vi "USBCool.vi"() -> ()   [LabVIEW 2015]
panel:
  out "Set Gate Mode":u32
  out "Shut Down":u32
  out "Cooler OFF":u32
  out "Detector Y Pixels":i32
  out "Get Detector":u32
  out "Get Status":u32
  out "Get Temperature":u32
  out "Cooler ON":u32
  out "Set Exposure Time":u32
  out "Set Trigger Mode":u32
  out "Set Readout Mode":u32
  out "Set Acquisition Mode":u32
  out "Current Temperature":i32
  out "Set Temperature":u32
  in  "Temperature":i32
  out "Check Timings":u32
  out "Detector X Pixels":i32
  out "Status":u32
  out "Graphical Results":i32[](graph)
  out "Start Acquisition":u32
  out "Get Acquired Data":u32
  out "Calculated Exposure Value":sgl format="%.5f"
  in  "Exposure Time (secs)":sgl format="%.2f"
  out "Initialize":u32
  in  "Trigger":u32(ring) items=["Internal", "External"]
  # "Status"
  # "Return values"
  # "USB iStar COOL32at.VI"
  # "Acquisition Mode: Single Scan\nReadout Mode: Full Vertical Binning\nCools to desired temperature, acquires data and then brings the temperature up to 0 in a controlled way."
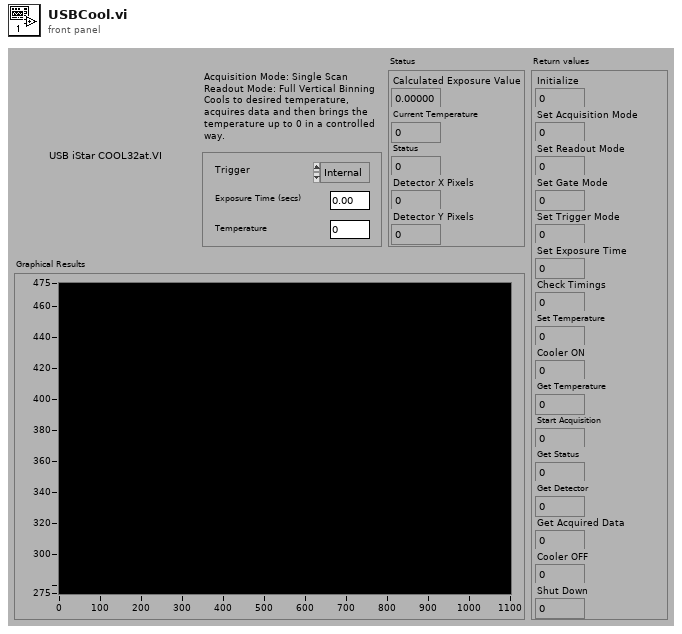
[diagram p1: front panel]
types:
  T1 = typedef "Error Code Enum typedef.ctl" = enum32{"N/A (0)", "DRV_ERROR_CODES", "DRV_SUCCESS", "DRV_VXDNOTINSTALLED", "DRV_ERROR_SCAN", "DRV_ERROR_CHECK_SUM", "DRV_ERROR_FILELOAD", "DRV_UNKNOWN_FUNC", "DRV_ERROR_VXD_INIT", "DRV_ERROR_ADDRESS", "DRV_ERROR_PAGELOCK", "DRV_ERROR_PAGEUNLOCK", "DRV_ERROR_BOARDTEST", "DRV_ERROR_ACK", "DRV_ERROR_UP_FIFO", "DRV_ERROR_PATTERN", "N/A (16)", "DRV_ACQUISITION_ERRORS", "DRV_ACQ_BUFFER", "DRV_ACQ_DOWNFIFO_FULL", "DRV_PROC_UNKONWN_INSTRUCTION", "DRV_ILLEGAL_OP_CODE", "DRV_KINETIC_TIME_NOT_MET", "DRV_ACCUM_TIME_NOT_MET", "DRV_NO_NEW_DATA", "N/A (25)", "DRV_SPOOLERROR", "N/A (27)", "N/A (28)", "N/A (29)", "N/A (30)", "N/A (31)", "N/A (32)", "DRV_TEMPERATURE_CODES", "DRV_TEMPERATURE_OFF", "DRV_TEMPERATURE_NOT_STABILIZED", "DRV_TEMPERATURE_STABILIZED", "DRV_TEMPERATURE_NOT_REACHED", "DRV_TEMPERATURE_OUT_RANGE", "DRV_TEMPERATURE_NOT_SUPPORTED", "DRV_TEMPERATURE_DRIFT", "N/A (41)", "N/A (42)", "N/A (43)", "N/A (44)", "N/A (45)", "N/A (46)", "N/A (47)", "N/A (48)", "DRV_GENERAL_ERRORS", "DRV_INVALID_AUX", "DRV_COF_NOTLOADED", "DRV_FPGAPROG", "DRV_FLEXERROR", "DRV_GPIBERROR", "N/A (55)", "N/A (56)", "N/A (57)", "N/A (58)", "N/A (59)", "N/A (60)", "N/A (61)", "N/A (62)", "N/A (63)", "DRV_DATATYPE", "DRV_DRIVER_ERRORS", "DRV_P1INVALID", "DRV_P2INVALID", "DRV_P3INVALID", "DRV_P4INVALID", "DRV_INIERROR", "DRV_COFERROR", "DRV_ACQUIRING", "DRV_IDLE", "DRV_TEMPCYCLE", "DRV_NOT_INITIALIZED", "DRV_P5INVALID", "DRV_P6INVALID", "DRV_INVALID_MODE", "DRV_INVALID_FILTER", "DRV_I2CERRORS", "DRV_I2CDEVNOTFOUND", "DRV_I2CTIMEOUT", "DRV_P7INVALID", "N/A (84)", "N/A (85)", "N/A (86)", "N/A (87)", "N/A (88)", "N/A (89)", "DRV_IOCERROR", "DRV_VRMVERSIONERROR"}
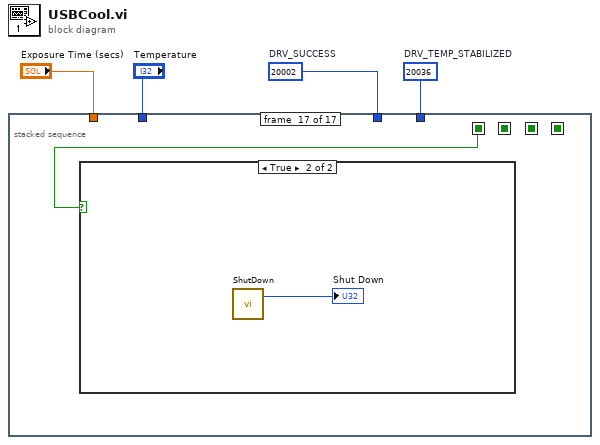
[diagram p0: block diagram]
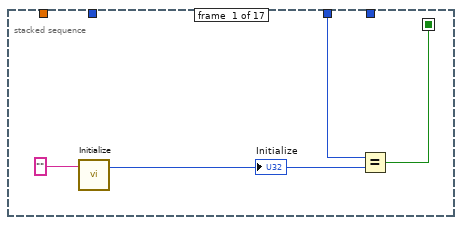
[diagram p2: hidden frame]
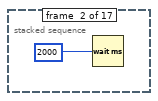
[diagram p3: hidden frame]
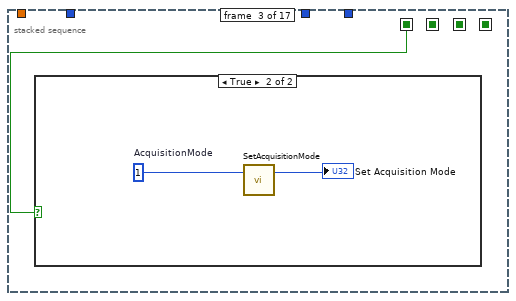
[diagram p4: hidden frame]
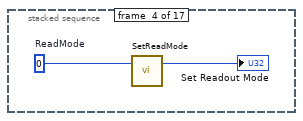
[diagram p6: hidden frame]
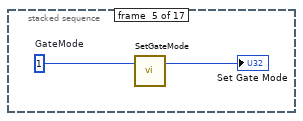
[diagram p7: hidden frame]
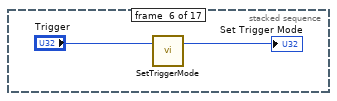
[diagram p8: hidden frame]
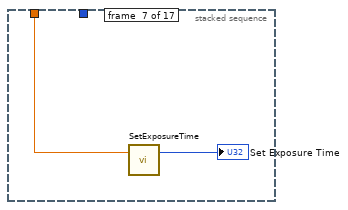
[diagram p9: hidden frame]
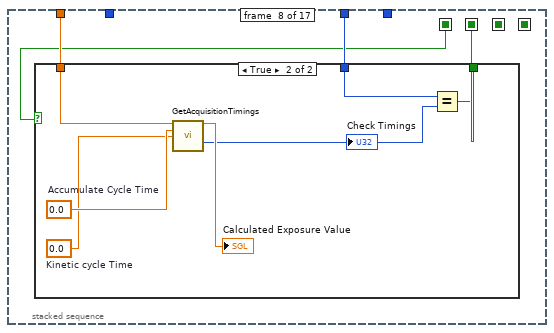
[diagram p10: hidden frame]
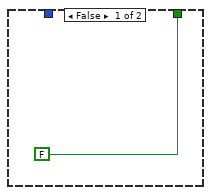
[diagram p11: hidden frame]
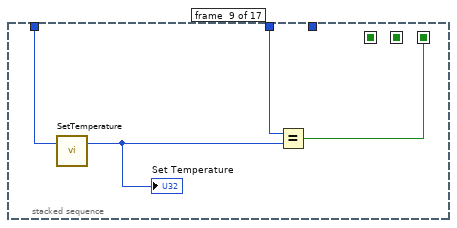
[diagram p12: hidden frame]
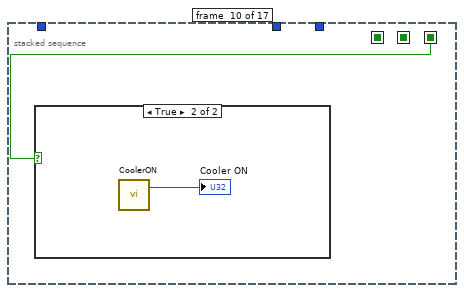
[diagram p13: hidden frame]
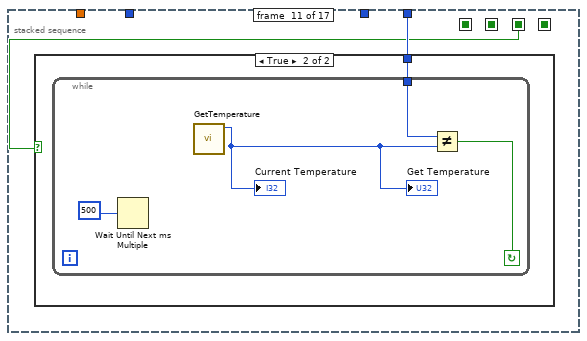
[diagram p15: hidden frame]
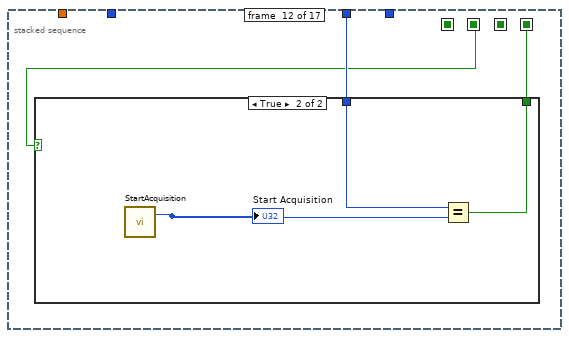
[diagram p17: hidden frame]
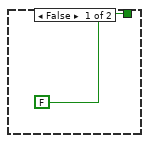
[diagram p18: hidden frame]
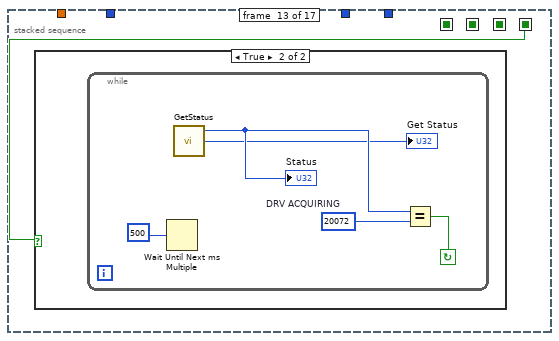
[diagram p19: hidden frame]
diagram:
  w1 = 20036  # DRV_TEMP_STABILIZED
  w3 = 20002  # DRV_SUCCESS
  n1 = stacked-sequence {
    seq-local: [w7 _ _ _ _ _ _ _ _ _ _ _ _ _ _ _ _] -> [_ _ w10 _ _ _ _ w21 _ _ _ _ _ _ _ _ w69]
    seq-local: [_ _ _ _ _ _ _ w22 _ _ _ _ _ _ _ _ _] -> [_ _ _ _ _ _ _ _ _ _ _ w47 _ _ _ _ _]
    seq-local: [_ _ _ _ _ _ _ _ _ _ _ w46 _ _ _ _ _] -> [_ _ _ _ _ _ _ _ _ _ _ _ w53 _ _ _ _]
    seq-local: [_ _ _ _ _ _ _ _ w35 _ _ _ _ _ _ _ _] -> [_ _ _ _ _ _ _ _ _ w37 w39 _ _ _ _ w64 _]
    tunnel: "Exposure Time (secs)" -> [_ _ _ _ _ _ w19 w24 _ _ _ _ _ _ _ _ _]
    tunnel: w3 -> [w8 _ _ _ _ _ _ w23 w36 _ _ w48 _ _ _ _ _]
    tunnel: "Temperature" -> [_ _ _ _ _ _ _ _ w34 _ _ _ _ _ _ _ _]
    tunnel: w1 -> [_ _ _ _ _ _ _ _ _ _ w40 _ _ _ _ _ _]
    frame #0 {
      n2 = call "Initialize.vi"("directory (\"\")"="") -> ("DLL error code"=w5:u32)  [unwired: 1 in, 1 out]
      "Initialize" <- w5
      n3 = Equal?(x=w8, y=w5) -> (x = y?=w7:bool)
    }
    frame #1 {
      n4 = Wait (ms)(milliseconds to wait=u32 2000) -> ()  [unwired: 1 out]
    }
    frame #2 {
      n5 = case shown="True" w10 {
        frame False {
        }
        frame True {
          w12 = u16 1  # AcquisitionMode
          n6 = call "SetAcquisitionMode.vi"("mode"=w12) -> ("DLL error code"=→"Set Acquisition Mode":u32)  [unwired: 1 in, 1 out]
        }
      }
    }
    frame #3 {
      w14 = u16 0  # ReadMode
      n7 = call "SetReadMode.vi"("mode"=w14) -> ("DLL error code"=→"Set Readout Mode":u32)  [unwired: 1 in, 1 out]
    }
    frame #4 {
      w15 = u16 1  # GateMode
      n8 = call "SetGateMode.vi"("mode"=w15) -> ("DLL error code"=→"Set Gate Mode":u32)  [unwired: 1 in, 1 out]
    }
    frame #5 {
      n9 = call "SetTriggerMode.vi"("mode"="Trigger") -> ("DLL error code"=→"Set Trigger Mode":u32)  [unwired: 1 in, 1 out]
    }
    frame #6 {
      n10 = call "SetExposureTime.vi"("time"=w19) -> ("DLL error code"=→"Set Exposure Time":u32)  [unwired: 1 in, 1 out]
    }
    frame #7 {
      n11 = case shown="True" w21 {
        tunnel: w24 -> [_ w30]
        tunnel: w23 -> [_ w31]
        tunnel: [FALSE w32] -> w22
        frame False {
        }
        frame True {
          w29 = sgl 0.0  # Accumulate Cycle Time
          w28 = sgl 0.0  # Kinetic cycle Time
          n12 = call "GetAcquisitionTimings.vi"("exposure input"=w30, "accumulate input"=w29, "kinetic input"=w28) -> ("exposure"=→"Calculated Exposure Value":sgl, "DLL error code"=w26:u32)  [unwired: 8 in, 3 out]
          "Check Timings" <- w26
          n13 = Equal?(x=w31, y=w26) -> (x = y?=w32:bool)
        }
      }
    }
    frame #8 {
      n14 = call "SetTemperature.vi"("temperature"=w34) -> ("DLL error code"=w33:u32)  [unwired: 1 in, 1 out]
      "Set Temperature" <- w33
      n15 = Equal?(x=w36, y=w33) -> (x = y?=w35:bool)
    }
    frame #9 {
      n16 = case shown="True" w37 {
        frame False {
        }
        frame True {
          n17 = call "CoolerON.vi"() -> ("DLL error code"=→"Cooler ON":u32)  [unwired: 2 in, 1 out]
        }
      }
    }
    frame #10 {
      n18 = case shown="True" w39 {
        tunnel: w40 -> [_ w41]
        frame False {
        }
        frame True {
          n19 = while {
            tunnel: w41 -> [w43]
            stop <- w44 continue-if-true
            n20 = Wait Until Next ms Multiple(millisecond multiple=u32 500) -> ()  [unwired: 1 out]
            n21 = call "GetTemperature.vi"() -> ("temperature"=w42:i32)  [unwired: 4 in, 3 out]
            "Current Temperature" <- w42
            "Get Temperature" <- w42
            n22 = Not Equal?(x=w43, y=w42) -> (x != y?=w44:bool)
          }
        }
      }
    }
    frame #11 {
      n23 = case shown="True" w47 {
        tunnel: [FALSE w52] -> w46
        tunnel: w48 -> [_ w51]
        frame False {
        }
        frame True {
          n24 = call "StartAcquisition.vi"() -> ("DLL error code"=w50:u32)  [unwired: 2 in, 1 out]
          "Start Acquisition" <- w50
          n25 = Equal?(x=w51, y=w50) -> (x = y?=w52:bool)
        }
      }
    }
    frame #12 {
      n26 = case shown="True" w53 {
        frame False {
        }
        frame True {
          n27 = while {
            stop <- w57 continue-if-true
            w56 = u16 20072  # DRV ACQUIRING
            n28 = Wait Until Next ms Multiple(millisecond multiple=u32 500) -> ()  [unwired: 1 out]
            n29 = call "GetStatus.vi"() -> ("DLL error code"=→"Get Status":u32, "status"=w55:T1)  [unwired: 3 in, 1 out]
            "Status" <- w55
            n30 = Equal?(x=w55, y=w56) -> (x = y?=w57:bool)
          }
        }
      }
    }
    frame #13 {
      n31 = call "GetDetector.vi"() -> ("ypixels"=→"Detector Y Pixels":i32, "xpixels"=w59:i32)  [unwired: 4 in, 2 out]
      "Detector X Pixels" <- w59
      "Get Detector" <- w59
      n32 = property on="Graphical Results" class="WFGraph (strict)"("X Scale.Range:Maximum"=w59) -> ()  [unwired: 2 in, 2 out]
      n33 = call "GetAcquiredData.vi"("size"=w59) -> ("DLL error code"=→"Get Acquired Data":u32, "array"=→"Graphical Results":i32[])  [unwired: 2 in, 1 out]
    }
    frame #14 {
      n34 = call "CoolerOFF.vi"() -> ("DLL error code"=→"Cooler OFF":u32)  [unwired: 2 in, 1 out]
    }
    frame #15 {
      n35 = case shown="True" w64 {
        frame False {
        }
        frame True {
          n36 = while {
            stop <- w66 continue-if-true
            n37 = Wait Until Next ms Multiple(millisecond multiple=u32 500) -> ()  [unwired: 1 out]
            n38 = call "GetTemperature.vi"() -> ("temperature"=w65:i32)  [unwired: 4 in, 3 out]
            n39 = local write "Current Temperature"(w65) -> ()
            n40 = Less?(x=w65, y=i16 0) -> (x < y?=w66:bool)
          }
        }
      }
    }
    frame #16 {
      n41 = case shown="True" w69 {
        frame False {
        }
        frame True {
          n42 = call "ShutDown.vi"() -> ("DLL error code"=→"Shut Down":u32)  [unwired: 2 in, 1 out]
        }
      }
    }
  }
